vi "4 Axis - Set Position.vi"(4 "error in (no error)":errorcluster, 7 "Controller Reference In":refnum<k7>) -> (0 "error out":errorcluster, 3 "Controller Reference Out":refnum<k7>)   [LabVIEW 2015]
doc: "Resets all 4 axis' position to zero."
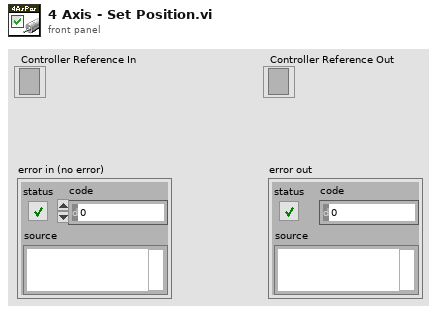
[diagram p1: front panel]
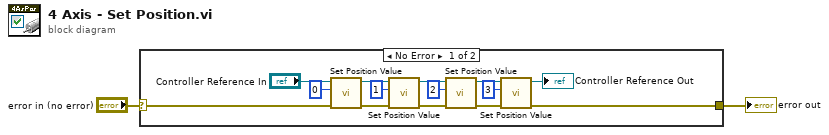
[diagram p0: block diagram]
diagram:
  n1 = case shown="No Error" "error in (no error)" {
    selector: "error in (no error)" -> [w15 w17]
    tunnel: [w6 w17] -> w2
    frame No Error {
      n2 = call "Set Position Value.vi"("error in (no error)"=w15, "Axis In"=i16 0, "Controller Reference"="Controller Reference In") -> ("error out"=w9:errorcluster, "Controller Reference out"=w13:refnum<k7>)  [unwired: 2 in, 1 out]
      n3 = call "Set Position Value.vi"("error in (no error)"=w9, "Axis In"=i16 1, "Controller Reference"=w13) -> ("error out"=w8:errorcluster, "Controller Reference out"=w12:refnum<k7>)  [unwired: 2 in, 1 out]
      n4 = call "Set Position Value.vi"("error in (no error)"=w8, "Axis In"=i16 2, "Controller Reference"=w12) -> ("error out"=w7:errorcluster, "Controller Reference out"=w11:refnum<k7>)  [unwired: 2 in, 1 out]
      n5 = call "Set Position Value.vi"("error in (no error)"=w7, "Axis In"=i16 3, "Controller Reference"=w11) -> ("error out"=w6:errorcluster, "Controller Reference out"=→"Controller Reference Out":refnum<k7>)  [unwired: 2 in, 1 out]
    }
    frame Error {
    }
  }
  "error out" <- w2
